vi "example_03_scrollbar.vi"() -> ()   [LabVIEW 2015, in "lv-graph-global.lvlib"]
uses:
  lv-graph-global.lvlib
  _controls/configuration.ctl
  _controls/store_method.ctl
  advanced/write-point.vi
  advanced/read-index.vi
  advanced/read-data.vi
  <userlib>/antonio-alexander/lv-graph/public/advanced/build_graph-single_axis.vi
  <userlib>/antonio-alexander/lv-graph/lv-graph.lvlib
panel:
  in  "points_to_generate":i32=5000
  in  "realtime":bool
  out "all_points_generated":bool
  in  "horizontal_scrollbar":i32(c297)
  in  "data_rate_ms":u32=10
  in  "refresh_rate_ms":i32=250
  in  "stop":bool
  out "horizontal_graph":T1(graph)
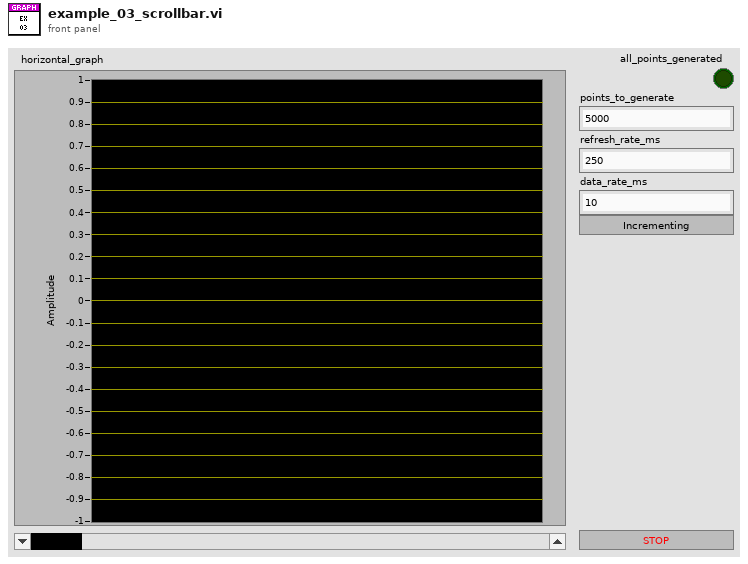
[diagram p1: front panel]
types:
  T1 = cluster{"Time [] out":dbl[], "Data[][] out":dbl[]}[]
  T2 = typedef "lv-graph-global.lvlib/configuration.ctl" = cluster{"store_method":T3, "rows":i32, "columns":i32}
  T3 = typedef "lv-graph-global.lvlib/store_method.ctl" = enum16{"<store_method>", "fixed", "grow"}
  T4 = cluster{"x_scale_maximum":dbl, "x_scale_minimum":dbl, "y_scale_maximum":dbl, "y_scale_minimum":dbl}
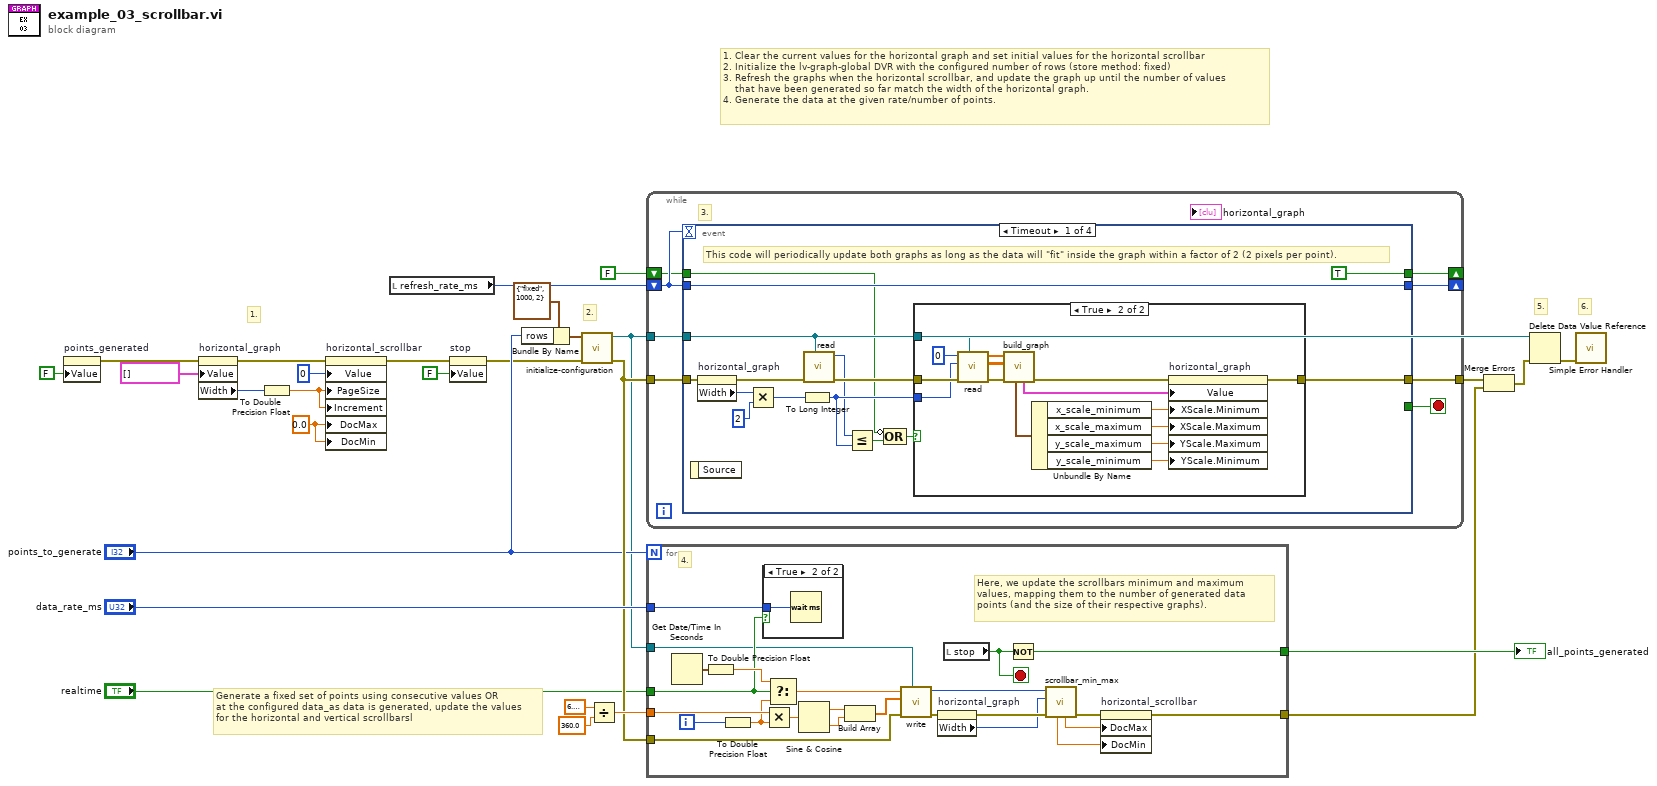
[diagram p0: block diagram]
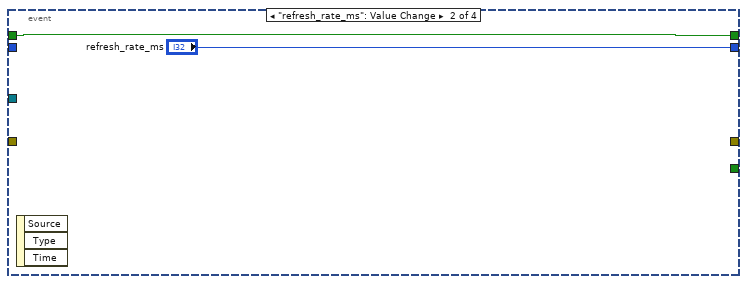
[diagram p3: hidden frame]
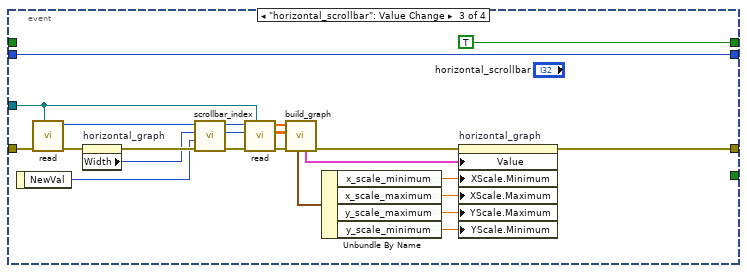
[diagram p4: hidden frame]
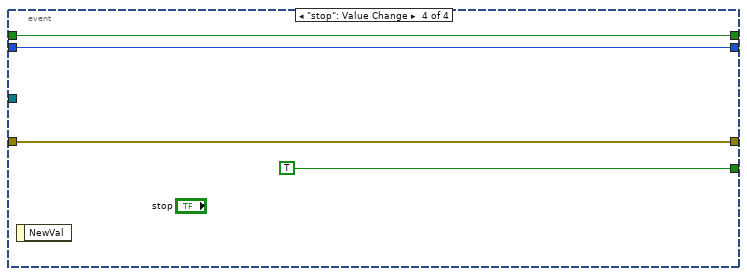
[diagram p5: hidden frame]
diagram:
  w22 = 0.0 ("Doc Max")
  # "1. Clear the current values for the horizontal graph and set initial values for the horizontal scrollbar\n2. Initialize the lv-graph-global DVR with the configured number of rows (store method: fixed)\n3. Refresh the graphs when the horizontal scrollbar, and update the graph up until the number of values\n    that have been generated so far match the width of the horizontal graph.\n4. Generate the data at the given rate/number of points."
  # "Generate a fixed set of points using consecutive values OR\nat the configured data_as data is generated, update the values\nfor the horizontal and vertical scrollbarsl"
  # "6."
  # "5."
  # "2."
  # "1."
  n1 = property on="points_generated" class="Bool (strict)"("Value"=FALSE ("All Points Generated?")) -> (error out=w15:errorcluster)  [unwired: 2 in, 1 out]
  n2 = property on="horizontal_graph" class="XYGraph (strict)"(error in=w15, "Value"=T1 [] ("Graph")) -> (error out=w23:errorcluster, "Width"=w21:u32)  [unwired: 1 in, 1 out]
  n3 = To Double Precision Float(number=w21) -> (double precision float=w13:dbl)
  n4 = property on="horizontal_scrollbar" class="Scroll (strict)"(error in=w23, "Value"=0 ("Scrollbar"), "PageSize"=w13, "Increment"=w13, "DocMax"=w22, "DocMin"=w22) -> (error out=w1:errorcluster)  [unwired: 1 in, 1 out]
  n5 = local read "refresh_rate_ms"() -> (w12:i32)
  n6 = property on="stop" class="Bool (strict)"(error in=w1, "Value"=FALSE ("Stop")) -> (error out=w5:errorcluster)  [unwired: 1 in, 1 out]
  n7 = Bundle By Name(cluster=T2 {"store_method"=enum."fixed", "rows"=1000, "columns"=2} ("configuration"), "rows"="points_to_generate") -> (w8:T2)
  n8 = call "initialize-configuration.vi"("error in (no error)"=w5, "configuration"=w8) -> ("error out"=w11:errorcluster, "dvr"=w6:refnum<data-value>)  [unwired: 8 in]
  n9 = Divide(x=6.283185307179586, y=360.0) -> (x/y=w17:dbl)
  n10 = while {
    tunnel: w11 -> [w36]
    tunnel: [w34] -> w28
    tunnel: w6 -> [w33]
    shift-right: [w31] -> _
    shift-left: w12 -> [w32]
    shift-right: [w29] -> _
    shift-left: FALSE -> [w30]
    stop <- w35 stop-if-true
    # "3."
    n11 = event shown="[0] Timeout" {
      selector: _ -> [_ _ _ _]
      dyn-events: _ -> [_ _ _ _]
      timeout: w32 -> [_ _ _ _]
      tunnel: w36 -> [w49 _ w88 w95]
      tunnel: [_ _ _ TRUE] -> w35
      tunnel: [w37 _ w87 w95] -> w34
      tunnel: w33 -> [w43 _ w73 _]
      tunnel: w32 -> [w44 _ w84 w94]
      tunnel: [w44 "refresh_rate_ms" w84 w94] -> w31
      tunnel: w30 -> [w38 w68 _ w93]
      tunnel: [TRUE w68 TRUE w93] -> w29
      event Timeout {
        # "This code will periodically update both graphs as long as the data will \"fit\" inside the graph within a factor of 2 (2 pixels per point)."
        n12 = event-data() -> ()  [unwired: 1 in, 1 out]
        n13 = property on="horizontal_graph" class="XYGraph (strict)"(error in=w49) -> (error out=w47:errorcluster, "Width"=w50:u32)  [unwired: 1 in, 1 out]
        n14 = Multiply(x=w50, y=u32 2 ("x")) -> (x*y=w48:u32)
        n15 = To Long Integer(number=w48) -> (32bit integer=w45:i32)
        n16 = call-poly "read.vi"("dvr"=w43, "error in (no error)"=w47) -> ("error out"=w46:errorcluster, "index"=w42:i32)  [unwired: 8 in]
        n17 = Less Or Equal?(x=w42, y=w45) -> (x <= y?=w40:bool)
        n18 = Compound Arithmetic op=OR(invert w38, w40) -> (w39:bool)
        n19 = case shown="True" w39 {
          tunnel: w46 -> [w52 w62]
          tunnel: [w52 w60] -> w37
          tunnel: w45 -> [_ w58]
          tunnel: w43 -> [_ w53]
          frame False {
          }
          frame True {
            n20 = call-poly "read.vi"("dvr"=w53, "error in (no error)"=w62, "length"=w58, "index in"=0 ("Index in")) -> ("error out"=w61:errorcluster, "y_axis"=w54:dbl[][], "x_axis"=w55:dbl[])  [unwired: 4 in, 1 out]
            n21 = call-poly <userlib>:"build_graph.vi"("error in (no error)"=w61, "y_axis"=w54, "x_axis"=w55) -> ("error out"=w67:errorcluster, "graph_data"=w56:cluster{dbl[], dbl[]}[], "scale_ranges"=w57:T4)  [unwired: 6 in]
            n22 = Unbundle By Name(w57) -> ("x_scale_minimum"=w65:dbl, "x_scale_maximum"=w66:dbl, "y_scale_maximum"=w64:dbl, "y_scale_minimum"=w63:dbl)
            n23 = property on="horizontal_graph" class="XYGraph (strict)"(error in=w67, "Value"=w56, "XScale.Minimum"=w65, "XScale.Maximum"=w66, "YScale.Maximum"=w64, "YScale.Minimum"=w63) -> (error out=w60:errorcluster)  [unwired: 1 in, 1 out]
          }
        }
      }
      event "refresh_rate_ms": Value Change {
        n24 = event-data() -> ()  [unwired: 1 in, 3 out]
      }
      event "horizontal_scrollbar": Value Change {
        n25 = event-data() -> ("NewVal"=w72:i32)  [unwired: 1 in]
        n26 = call-poly "read.vi"("dvr"=w73, "error in (no error)"=w88) -> ("error out"=w89:errorcluster, "index"=w71:i32)  [unwired: 8 in]
        n27 = property on="horizontal_graph" class="XYGraph (strict)"(error in=w89) -> (error out=w92:errorcluster, "Width"=w90:u32)  [unwired: 1 in, 1 out]
        n28 = call <userlib>:"scrollbar_index.vi"("error in (no error)"=w92, "seek"=w72, "width_height"=w90, "data_available"=w71) -> ("error out"=w85:errorcluster, "length"=w82:i32, "index"=w83:i32)  [unwired: 5 in]
        n29 = call-poly "read.vi"("dvr"=w73, "error in (no error)"=w85, "length"=w82, "index in"=w83) -> ("error out"=w86:errorcluster, "y_axis"=w80:dbl[][], "x_axis"=w81:dbl[])  [unwired: 4 in, 1 out]
        n30 = call-poly <userlib>:"build_graph.vi"("error in (no error)"=w86, "y_axis"=w80, "x_axis"=w81) -> ("error out"=w91:errorcluster, "graph_data"=w78:cluster{dbl[], dbl[]}[], "scale_ranges"=w79:T4)  [unwired: 6 in]
        n31 = Unbundle By Name(w79) -> ("x_scale_minimum"=w77:dbl, "x_scale_maximum"=w76:dbl, "y_scale_maximum"=w75:dbl, "y_scale_minimum"=w74:dbl)
        n32 = property on="horizontal_graph" class="XYGraph (strict)"(error in=w91, "Value"=w78, "XScale.Minimum"=w77, "XScale.Maximum"=w76, "YScale.Maximum"=w75, "YScale.Minimum"=w74) -> (error out=w87:errorcluster)  [unwired: 1 in, 1 out]
      }
      event "stop": Value Change {
        n33 = event-data() -> ()  [unwired: 1 in, 1 out]
      }
    }
  }
  n34 = for {
    N: "points_to_generate" -> [_]
    tunnel: w17 -> [w118]
    tunnel: "realtime" -> [w106]
    tunnel: "data_rate_ms" -> [w107]
    tunnel: [w111] -> w19
    tunnel: w11 -> [w105]
    tunnel: [w97] -> w16
    tunnel: w6 -> [w98]
    i -> [w119]
    stop <- w112 stop-if-true
    # "Here, we update the scrollbars minimum and maximum\nvalues, mapping them to the number of generated data\npoints (and the size of their respective graphs)."
    # "4."
    n35 = Get Date/Time In Seconds() -> (seconds since 1Jan1904=w120:timestamp)
    n36 = To Double Precision Float(number=w120) -> (double precision float=w117:dbl)
    n37 = To Double Precision Float(number=w119) -> (double precision float=w116:dbl)
    n38 = case shown="True" w106 {
      tunnel: w107 -> [_ w121]
      frame False {
      }
      frame True {
        n39 = Wait (ms)(milliseconds to wait=w121) -> ()  [unwired: 1 out]
      }
    }
    n40 = Multiply(x=w118, y=w116) -> (x*y=w115:dbl)
    n41 = Select(t=w117, s=w106, f=w116) -> (s? t:f=w103:dbl)
    n42 = Sine & Cosine(0:w115) -> (1:w114:dbl, 2:w113:dbl)
    n43 = Build Array(w114, w113) -> (w102:dbl[])
    n44 = call-poly "write.vi"("dvr"=w98, "error in (no error)"=w105, "y_axis"=w102, "x_axis"=w103) -> ("error out"=w104:errorcluster, "index"=w101:i32)  [unwired: 6 in]
    n45 = property on="horizontal_graph" class="XYGraph (strict)"(error in=w104) -> (error out=w109:errorcluster, "Width"=w108:u32)  [unwired: 1 in, 1 out]
    n46 = local read "stop"() -> (w112:bool)
    n47 = Not(x=w112) -> (.not. x?=w111:bool)
    n48 = call <userlib>:"scrollbar_min_max.vi"("error in (no error)"=w109, "width_height"=w108, "data_index in"=w101) -> ("error out"=w110:errorcluster, "scrollbar_doc_max"=w99:dbl, "scrollbar_doc_min"=w100:dbl)  [unwired: 6 in]
    n49 = property on="horizontal_scrollbar" class="Scroll (strict)"(error in=w110, "DocMax"=w99, "DocMin"=w100) -> (error out=w97:errorcluster)  [unwired: 1 in, 1 out]
  }
  "all_points_generated" <- w19
  n50 = Merge Errors(w28, w16) -> (w9:errorcluster)
  n51 = Delete Data Value Reference(data value reference=w6, error in=w9) -> (error out=w4:errorcluster)  [unwired: 1 out]
  n52 = call <vilib>:"Simple Error Handler.vi"("error in (no error)"=w4) -> ()  [unwired: 4 in, 5 out]
